vi "注册.vi"() -> ()   [LabVIEW 2015]
uses:
  <vilib>/Utility/file.llb/Read Delimited Spreadsheet (string).vi
  <vilib>/Utility/file.llb/Write Delimited Spreadsheet (string).vi
panel:
  in  "关闭":bool
  in  "刷新按钮":bool
  in  "用户信息":string[][](array[string]) caption="所有行"
  # "用户名"
  # "密码"
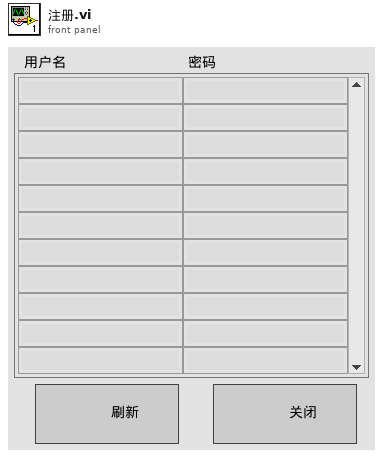
[diagram p1: front panel]
types:
  T1 = enum16{"open", "replace", "create", "open or create", "replace or create", "replace or create with confirmation"}
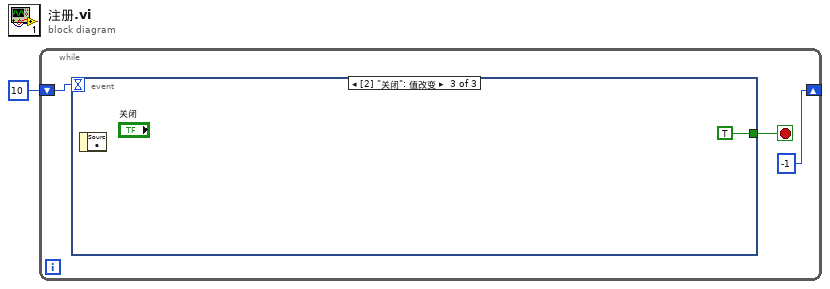
[diagram p0: block diagram]
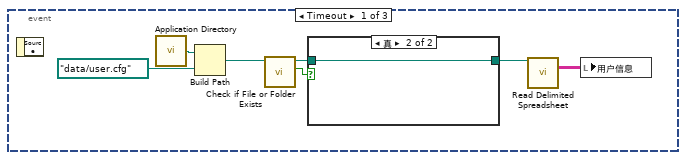
[diagram p2: hidden frame]
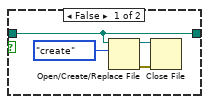
[diagram p3: hidden frame]
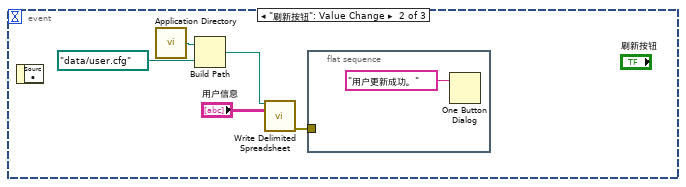
[diagram p4: hidden frame]
diagram:
  n1 = while {
    shift-right: [-1] -> _
    shift-left: 10 -> [w4]
    stop <- w2 stop-if-true
    n2 = event shown="[2] \"关闭\": 值改变" {
      selector: _ -> [_ _ _]
      dyn-events: _ -> [_ _ _]
      timeout: w4 -> [_ _ _]
      tunnel: [_ _ TRUE] -> w2
      event Timeout {
        n3 = event-data() -> ()  [unwired: 1 in, 1 out]
        n4 = call <vilib>:"Application Directory.vi"() -> ("Application Directory"=w10:path)
        n5 = Build Path(base path=w10, name or relative path=path "data/user.cfg") -> (appended path=w9:path)
        n6 = call <vilib>:"Check if File or Folder Exists.vi"("path"=w9) -> ("file or folder exists?"=w8:bool, "dup path"=w7:path)  [unwired: 8 in, 1 out]
        n7 = case shown="真" w8 {
          tunnel: w7 -> [w12 w16]
          tunnel: [w12 w16] -> w5
          frame False {
            n8 = Open/Create/Replace File(file path (use dialog)=w12, operation (0:open)=T1."create" ("操作(0:open)")) -> (refnum out=w13:refnum<file>, error out=w14:errorcluster)  [unwired: 4 in, 1 out]
            n9 = Close File(refnum=w13, error in=w14) -> ()  [unwired: 2 out]
          }
          frame True {
          }
        }
        n10 = call-poly <vilib>:"Read Delimited Spreadsheet.vi"("file path (dialog if empty)"=w5) -> ("all rows"=w6:string[][])  [unwired: 9 in, 5 out]
        n11 = local write "用户信息"(w6) -> ()
      }
      event "刷新按钮": Value Change {
        n12 = event-data() -> ()  [unwired: 1 in, 1 out]
        n13 = call <vilib>:"Application Directory.vi"() -> ("Application Directory"=w20:path)
        n14 = Build Path(base path=w20, name or relative path=path "data/user.cfg") -> (appended path=w19:path)
        n15 = call-poly <vilib>:"Write Delimited Spreadsheet.vi"("file path (dialog if empty)"=w19, "2D data"="用户信息") -> ("error out"=w17:errorcluster)  [unwired: 12 in, 1 out]
        n16 = flat-sequence {
          tunnel: w17 -> [_]
          frame #0 {
            n17 = One Button Dialog(message="用户更新成功。" ("消息")) -> ()  [unwired: 1 in, 1 out]
          }
        }
      }
      event "关闭": Value Change {
        n18 = event-data() -> ()  [unwired: 1 in, 1 out]
      }
    }
  }
